vi "Configure Device.vi"(8 "error in (no error)":errorcluster, 10 "Max beams":dbl, 11 "Device-Thru in":refnum<class "Thru.lvclass">) -> (0 "error out":errorcluster, 3 "Device-Thru out":refnum<class "Thru.lvclass">)   [LabVIEW 2020, in "Thru.lvclass"]
doc: "Interface for configuring the device for testing"
uses:
  Thru.lvclass
  C:/Sandbox/Git_Sandbox/WiSpry Test Framework source code (LV20)/WiSpry Test Framework/Devices/Device.lvclass
  Controls/Register to Write.ctl
  PIC-device/PIC-Device.lvclass
panel:
  in  "OK Button":bool
  # "There is nothing to configure"
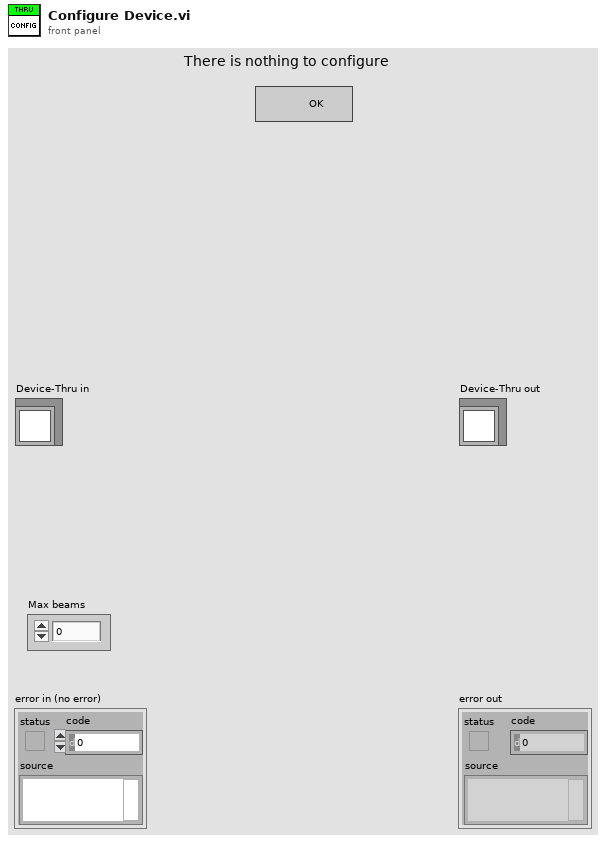
[diagram p1: front panel]
types:
  T1 = typedef "PIC-Device.lvclass/Register to Write.ctl" = cluster{"Register":u32, "Value":u32, "Dev Address":u32, "Physical Adress":u32}
  T2 = typedef "Device.lvclass/Device Information Cluster.ctl" = cluster{"Device Info":string[][], "Default Values":T1[], "Fetched info":string[][]}
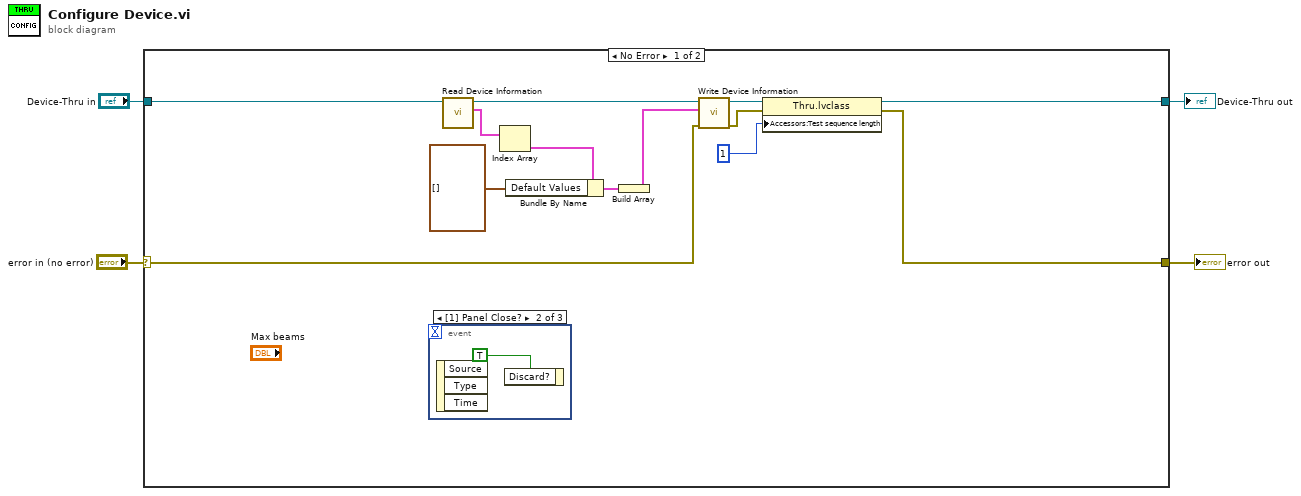
[diagram p0: block diagram]
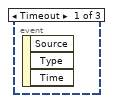
[diagram p2: hidden frame]
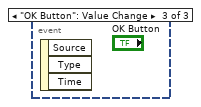
[diagram p3: hidden frame]
diagram:
  n1 = case shown="No Error" "error in (no error)" {
    selector: "error in (no error)" -> [w7 w20]
    tunnel: "Device-Thru in" -> [w12 w19]
    tunnel: [w6 w20] -> w2
    tunnel: [w5 w19] -> w1
    frame No Error {
      n2 = event shown="[1] Panel Close?" {
        selector: _ -> [_ _ _]
        dyn-events: _ -> [_ _ _]
        timeout: _ -> [_ _ _]
        event Timeout {
          n3 = event-data() -> ()  [unwired: 1 in, 3 out]
        }
        event Panel Close? {
          n4 = event-data() -> ()  [unwired: 1 in, 3 out]
          n5 = event-data("Discard?"=TRUE) -> ()  [unwired: 1 in, 1 out]
        }
        event "OK Button": Value Change {
          n6 = event-data() -> ()  [unwired: 1 in, 3 out]
        }
      }
      n7 = call-dynamic "Read Device Information.vi"("Device in"=w12) -> ("Device Info"=w14:T2[], "Device out"=w11:refnum<class "Thru.lvclass">)  [unwired: 8 in, 1 out]
      n8 = Index Array(array=w14) -> (element=w13:T2)  [unwired: 1 in]
      n9 = Bundle By Name(cluster=w13, "Default Values"=T1[] []) -> (w16:T2)
      n10 = Build Array(w16) -> (w15:T2[])
      n11 = call-dynamic "Write Device Information.vi"("error in (no error)"=w7, "Device Info"=w15, "Device in"=w11) -> ("error out"=w8:errorcluster, "Device out"=w10:refnum<class "Thru.lvclass">)  [unwired: 7 in]
      n12 = property class="Thru.lvclass"(reference=w10, error in=w8, "Accessors:Test sequence length"=1 ("Test sequence length")) -> (reference out=w5:refnum<class "Thru.lvclass">, error out=w6:errorcluster)
    }
    frame Error {
    }
  }
  "error out" <- w2
  "Device-Thru out" <- w1
